vi "LVClass_CorrectionDataManager GetInteractionMatrixData.vi"(0 "CorrectionDataManager in":refnum<class "CorrectionDataManager.lvclass">, 11 "error in (no error)":errorcluster) -> (4 "CorrectionDataManager out":refnum<class "CorrectionDataManager.lvclass">, 6 "Interaction matrix":sgl[][](array[numeric]), 15 "error out":errorcluster)   [LabVIEW 2020, in "CorrectionDataManager.lvclass"]
doc: "Interaction matrix content getter.\n\n--------------------------------------------------------------------------------\n\n<B>corrdata_managerIn </B> : CorrDataManager object.\n<B>corrdata_managerOut </B> : CorrDataManager object.\n<B>data </B> : 2D Array of interaction matrix content.\n<B>ErrorIn </B> : Error\n<B>ErrorOut </B> : Error\n\n--------------------------------------------------------------------------------"
uses:
  CorrectionDataManager.lvclass
  CorrectionDataManager.lvclass/CorrectionDataManager.ctl
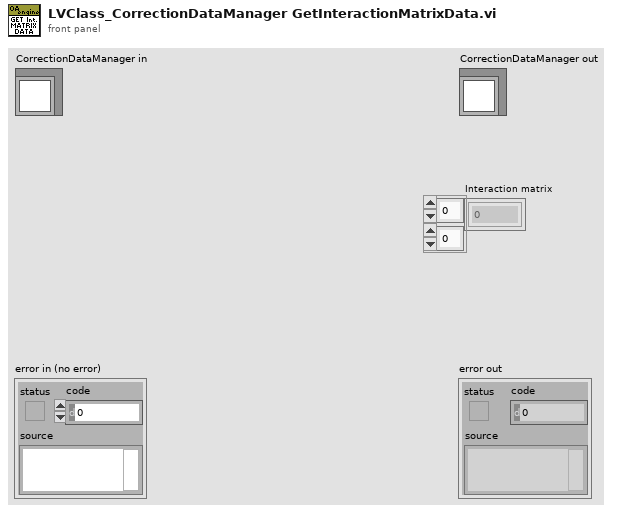
[diagram p1: front panel]
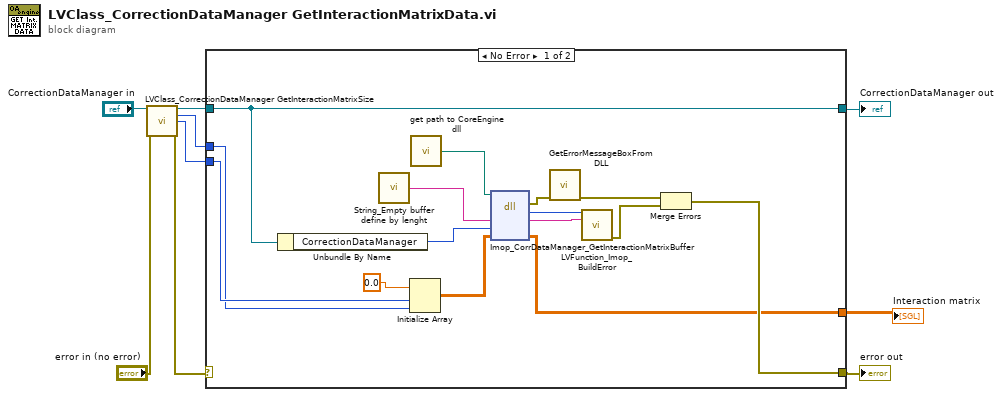
[diagram p0: block diagram]
diagram:
  n1 = call "LVClass_CorrectionDataManager GetInteractionMatrixSize.vi"("CorrectionDataManager in"="CorrectionDataManager in", "error in (no error)"="error in (no error)") -> ("CorrectionDataManager out"=w4:refnum<class "CorrectionDataManager.lvclass">, "# of valid actuators (nb col)"=w1:u32, "2 time of valid sub pupil (nb line)"=w3:u32, "error out"=w6:errorcluster)  [unwired: 10 in]
  n2 = case shown="No Error" w6 {
    selector: w6 -> [_ w26]
    tunnel: [w17 w26] -> w8
    tunnel: [w14 w25] -> w9
    tunnel: w4 -> [w14 w25]
    tunnel: w3 -> [w11 _]
    tunnel: [w12 _] -> w2
    tunnel: w1 -> [w10 _]
    frame No Error {
      n3 = Unbundle By Name(w14) -> ("CorrectionDataManager"=w16:i32)
      n4 = call "String_Empty buffer define by lenght.vi"() -> ("Empty buffer"=w22:string)  [unwired: 1 in]
      n5 = Initialize Array(sgl 0.0 ("Numeric"), w11, w10) -> (w13:sgl[][])
      n6 = call "get path to CoreEngine dll.vi"() -> ("path to c_interface_vc100.dll"=w21:path)  [unwired: 12 in, 3 out]
      n7 = dll-call lib="D:/soft/HASO_v3/SVN_trunk/ImOpCoreEngine4_LV2011/DLLs/c_interface_vc100.dll" fn="Imop_CorrDataManager_GetInteractionMatrixBuffer"(path in=w21, "message"=w22, "WavefrontCorrection"=w16, "Data Matrix"=w13) -> (error out=w20:errorcluster, "return type"=w24:i32, "message"=w23:string, "Data Matrix"=w12:sgl[][])  [unwired: 3 in, 1 out]
      n8 = call "GetErrorMessageBoxFromDLL.vi"("error IN"=w20) -> ("error OUT"=w19:errorcluster)  [unwired: 10 in]
      n9 = call "LVFunction_Imop_BuildError.vi"("code"=w24, "String to Prepend to source (\"\")"=w23) -> ("error out"=w18:errorcluster)  [unwired: 13 in]
      n10 = Merge Errors(w19, w18) -> (w17:errorcluster)
    }
    frame Error {
    }
  }
  "error out" <- w8
  "CorrectionDataManager out" <- w9
  "Interaction matrix" <- w2
